vi "Begin.vi"(8 "error in":errorcluster) -> (0 "error out":errorcluster)   [LabVIEW 2015]
doc: "Called before other user functions, this VI is expected to open initial I/O refnums, load in file data, and do all program initialization. Notice that the <B>error out</B> terminal is simply used for data flow. Wiring it to other structures or subVIs ensures that this VI runs first."
uses:
  <vilib>/Rock Robotics/SystemInterfaces/DIO/FPGA_DIOPWMChannel.ctl
  <vilib>/Rock Robotics/WPI/SafetyOutput/WPI_SafetyOutputConfigMenu.ctl
  <vilib>/Rock Robotics/WPI/DriverStation/WPI_DriverStationRobotMode2.ctl
  <vilib>/Rock Robotics/WPI/Joystick/WPI_JoystickDeviceEnum.ctl
  <vilib>/Rock Robotics/WPI/CAN/TalonSRX/WPI_CANTalonSRX_APIControlMode.ctl
  <vilib>/Rock Robotics/WPI/CAN/TalonSRX/WPI_CANTalonSRX_BrakeOverride.ctl
  <vilib>/Rock Robotics/WPI/CAN/TalonSRX/WPI_CANTalonSRX_APIFeedbackSelect.ctl
  <vilib>/Rock Robotics/WPI/CAN/TalonSRX/WPI_CANTalonSRX_Params.ctl
  <vilib>/Rock Robotics/WPI/RobotDrive/WPI_RobotDriveOpen2MotorWithTalon.vi
  Robot Global Data.vi
  <vilib>/Rock Robotics/Network Tables/NT Write String Array.vi
  <vilib>/Rock Robotics/WPI/MotorControl/WPI_MotorControlOpenCANTalonSRX.vi
panel:
  in  "Reverse Feedback Sensor":bool
  in  "Reverse Closed-Loop Output":bool
  in  "Maximum Output Voltage":dbl=12.0
  in  "Reverse Limit Position":dbl=-50.0
  in  "Forward Limit Position":dbl=50.0
  in  "Encoder Codes Per Rev":u16=2122
  in  "D":dbl=10.0
  in  "I":dbl=0.0001
  in  "P":dbl=0.4
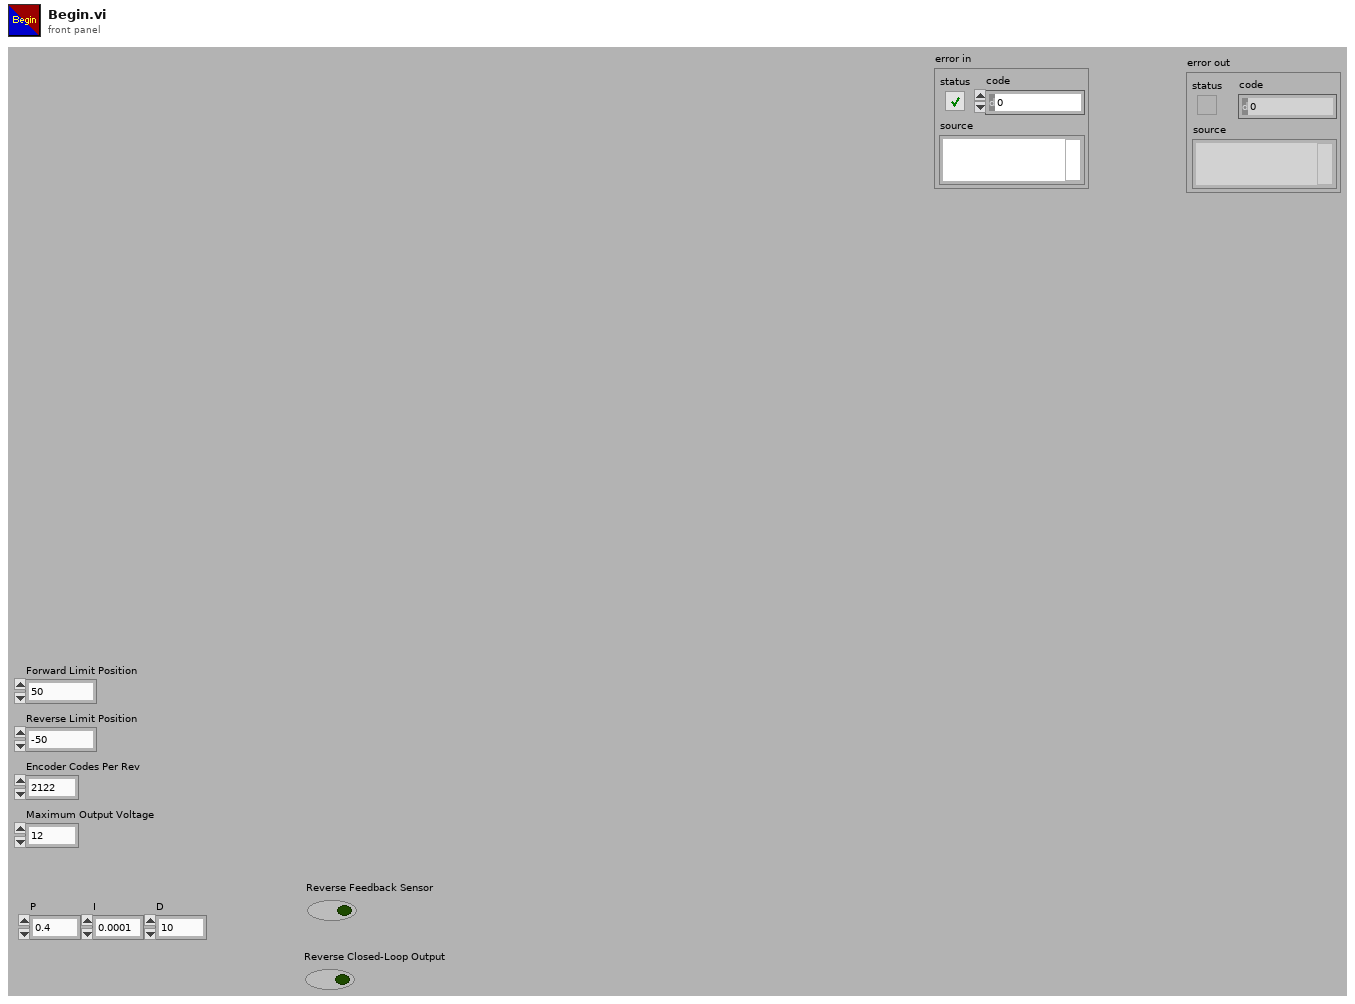
[diagram p1: front panel]
types:
  T1 = typedef "WPI_CANTalonSRX_APIControlMode.ctl" = enum8{"Percent VBus", "Speed", "Position", "Slave", "Unchanged / Invalid", "Voltage Compensation", "Current", "Motion Profile"}
  T2 = typedef "WPI_CANTalonSRX_Params.ctl" = u8
  T3 = typedef "WPI_CANTalonSRX_APIFeedbackSelect.ctl" = enum16{"Digital Quadrature Encoder", "Analog Potentiometer", "Analog Encoder", "Count on Quad-A (Rising-Edge)", "Count on Quad-A (Falling-Edge)", "CTR Magnetic Enc (Absolute)", "CTR Magnetic Enc (Relative)", "Pulse Width"}
  T4 = typedef "WPI_CANTalonSRX_BrakeOverride.ctl" = enum8{"No Override", "Override to Coast", "Override to Brake"}
  T5 = typedef "WPI_JoystickDeviceEnum.ctl" = enum16{"USB 0", "USB 1", "USB 2", "USB 3", "USB 4", "USB 5"}
  T6 = typedef "WPI_DriverStationRobotMode2.ctl" = enum16{"Autonomous Disabled", "Autonomous Enabled", "Teleop Disabled", "Teleop Enabled", "Disconnected", "Finish", "Test Disabled", "Test Enabled", "Emergency Stopped"}
  T7 = typedef "WPI_SafetyOutputConfigMenu.ctl" = enum16{"Enable", "Disable"}
  T8 = typedef "FPGA_DIOPWMChannel.ctl" = enum8{"PWM 0", "PWM 1", "PWM 2", "PWM 3", "PWM 4", "PWM 5", "PWM 6", "PWM 7", "PWM 8", "PWM 9", "PWM MXP 0", "PWM MXP 1", "PWM MXP 2", "PWM MXP 3", "PWM MXP 4", "PWM MXP 5", "PWM MXP 6", "PWM MXP 7", "PWM MXP 8", "PWM MXP 9", "Invalid"}
  T9 = typedef "WPI_MotorControlDeviceRef.ctl" = cluster{"DeviceStatus":errorcluster, "Type":T10, "PWM":cluster{"PWM Channel":T8, "DeadBand":T11}, "CAN":cluster{"Device Number":u8, "Control Mode":T12, "Semaphore":T13, "Max Vout":dbl, "TalonSRX Control Mode":T1}, "Invert":bool}
  T10 = typedef "WPI_MotorControlType.ctl" = enum16{"PWM", "CAN", "CANTalonSRX"}
  T11 = typedef "WPI_PWMDeadband.ctl" = cluster{"Name":string, "maxPositivePwm":i32, "minPositivePwm":i32, "centerPwm":i32, "maxNegativePwm":i32, "minNegativePwm":i32, "angularRange":u16}
  T12 = typedef "WPI_CANJaguar_ControlMode.ctl" = enum8{"Percent VBus", "Current", "Speed", "Position", "Voltage"}
  T13 = typedef "Semaphore RefNum" = refnum<k1>
  T14 = typedef "WPI_JoystickDevRef.ctl" = cluster{"Device":T5}
  T15 = typedef "WPI_RobotDriveDevRef.ctl" = cluster{"DevStatus":errorcluster, "Motors[]":T9[], "Square Inputs":bool, "Max Output":dbl}
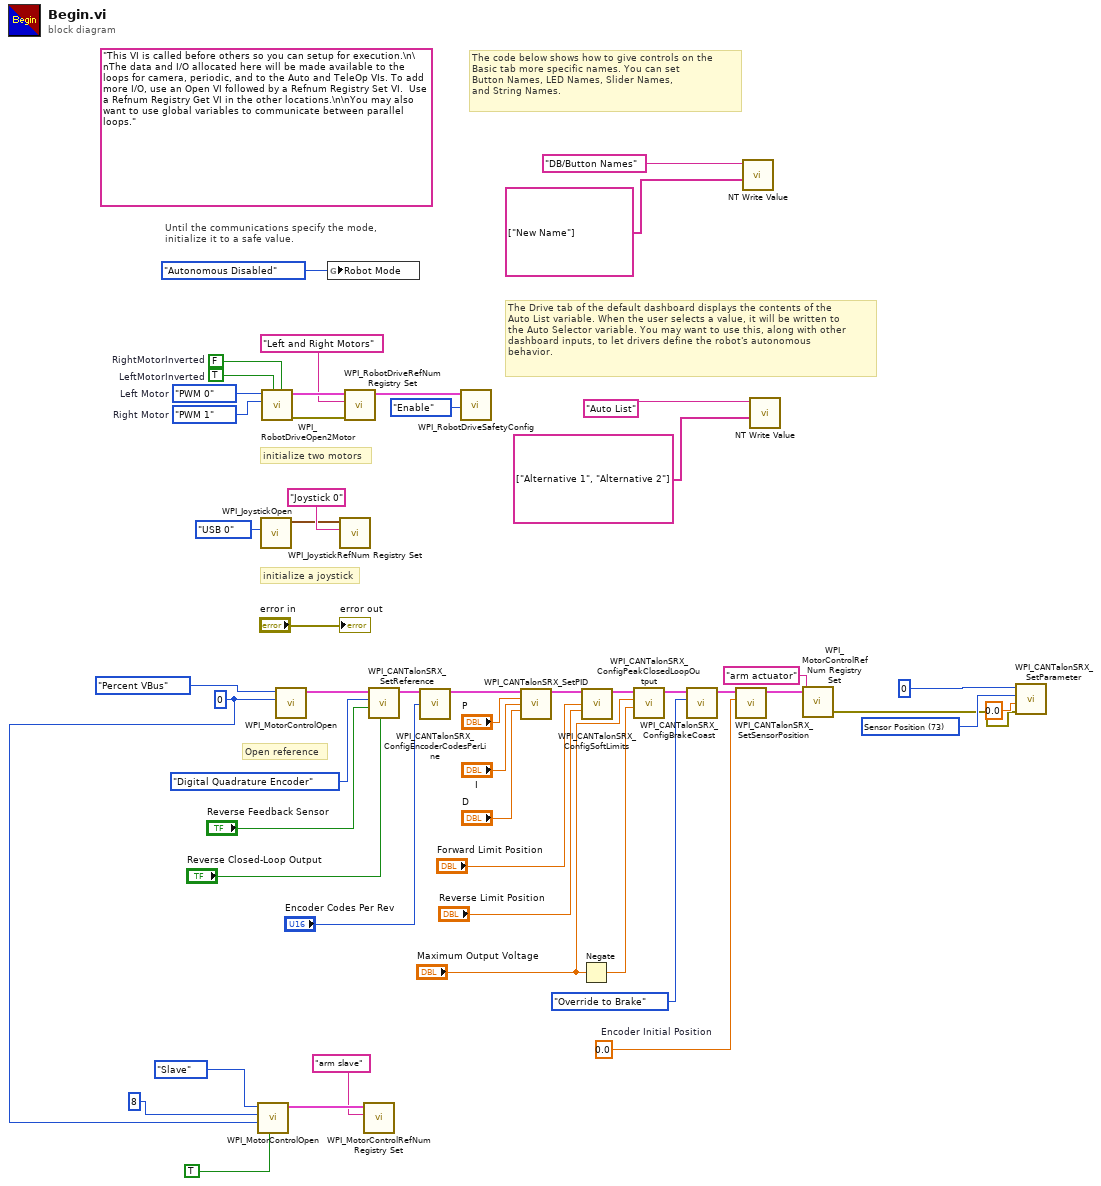
[diagram p0: block diagram]
diagram:
  w10 = T2 73 items=["Slot 0 - P"=1, "Slot 0 - I"=2, "Slot 0 - D"=3, "Slot 0 - F"=4, "Slot 0 - I Zone"=5, "Slot 0 - Ramp Rate"=6, "Slot 1 - P"=11, "Slot 1 - I"=12, "Slot 1 - D"=13, "Slot 1 - F"=14, "Slot 1 - I Zone"=15, "Slot 1 - Ramp Rate"=16, "Soft Limit - Forward"=21, "Soft Limit - Reverse"=22, "Soft Limit - Forward Enable"=23, "Soft Limit - Reverse Enable"=24, "On Boot - Brake Mode"=31, "On Boot - Limit Normally Closed - Forward"=32, "On Boot - Limit Normally Closed - Reverse"=33, "On Boot - Limit Disabled - Forward"=34, "On Boot - Limit Disabled - Reverse"=35, "Fault - Over Temp"=41, "Fault - Under Voltage"=42, "Fault - Forward Limit"=43, "Fault - Reverse Limit"=44, "Fault - Hardware Failure"=45, "Fault - Forward Soft Limit"=46, "Fault - Reverse Soft Limit"=47, "Sticky Fault - Over Temp"=48, "Sticky Fault - Under Voltage"=49, "Sticky Fault - Forward Limit"=50, "Sticky Fault - Reverse Limit"=51, "Sticky Fault - Forward Soft Limit"=52, "Sticky Fault - Reverse Soft Limit"=53, "Applied Throttle"=61, "Closed-Loop Error"=62, "Select Feedback Device"=63, "Reverse Closed-Loop Output"=64, "Mode Select"=65, "Profile Slot Select"=66, "Ramp Throttle"=67, "Reverse Feedback Sensor"=68, "Limit Switch Enabled"=69, "Limit Switch Closed - Forward"=70, "Limit Switch Closed - Reverse"=71, "Sensor Position"=73, "Sensor Velocity"=74, "Current"=75, "Brake is Enabled"=76, "Encoder Position"=77, "Encoder Velocity"=78, "Encoder Index Rise Events"=79, "Encoder A Pin State"=80, "Encoder B Pin State"=81, "Encoder Index Pin State"=82, "Analog In with Overflow"=83, "Analog In Velocity"=84, "Temperature"=85, "Battery Voltage"=86, "Reset Count"=87, "Reset Flags"=88, "Firmware Version"=89, "Settings Changed"=90, "Quad Filter Enable"=91, "Ignore Disable Broadcast"=92, "I Accumulator"=93, "Status 1 Frame Rate Ms"=94, "Status 2 Frame Rate Ms"=95, "Status 3 Frame Rate Ms"=96, "Status 4 Frame Rate Ms"=97, "Status 6 Frame Rate Ms"=98, "Status 7 Frame Rate Ms"=99, "Enable Index Pin Clear Position"=100, "Peak Positive Output"=104, "Nominal Positive Output"=105, "Peak Negative Output"=106, "Nominal Negative Output"=107, "Quad Index Pin Polarity"=108, "Status 8 Frame Rate Ms"=109, "Allow Position Overflow"=110, "Slot 0 - Allowable Closed-Loop Error"=111, "Number Potentiometer Turns"=112, "Encoder Codes Per Rev"=113, "Pulse Width Decoded Position"=114, "Analog Position"=115, "Voltage Compensation Rate (V/s)"=116, "Slot 1 - Allowable Closed-Loop Error"=117, "Motion Profile Has Underrun Err"=119] ("Parameter")
  w5 = u8 0 ("Device Number")
  w18 = 0.0  # Encoder Initial Position
  (unwired) "This VI is called before others so you can setup for execution.\n\nThe data and I/O allocated here will be made available to the loops for camera, periodic, and to the Auto and TeleOp VIs. To add more I/O, use an Open VI followed by a Refnum Registry Set VI.  Use a Refnum Registry Get VI in the other locations.\n\nYou may also want to use global variables to communicate between parallel loops."
  w45 = FPGA_DIOPWMChannel."PWM 1"  # Right Motor
  w46 = FPGA_DIOPWMChannel."PWM 0"  # Left Motor
  w50 = TRUE  # LeftMotorInverted
  w51 = FALSE  # RightMotorInverted
  # "Open reference"
  # "The Drive tab of the default dashboard displays the contents of the\nAuto List variable. When the user selects a value, it will be written to\nthe Auto Selector variable. You may want to use this, along with other\ndashboard inputs, to let drivers define the robot's autonomous\nbehavior."
  # "The code below shows how to give controls on the\nBasic tab more specific names. You can set\nButton Names, LED Names, Slider Names,\nand String Names."
  # "initialize a joystick"
  # "Until the communications specify the mode,\ninitialize it to a safe value."
  # "initialize two motors"
  n1 = call-poly <vilib>:"WPI_MotorControlOpen.vi"("Invert"=TRUE, "Master Device Number"=w5, "Device Number"=u8 8, "Control Mode"=WPI_CANTalonSRX_APIControlMode."Slave") -> ("MotorControlDeviceRef"=w2:T9)  [unwired: 1 in, 6 out]
  n2 = call <vilib>:"WPI_JoystickOpen.vi"("JoystickDevice"=WPI_JoystickDeviceEnum."USB 0") -> ("JoystickDevRef"=w40:T14)  [unwired: 10 in]
  n3 = call-poly <vilib>:"WPI_RobotDriveOpen2Motor.vi"("Right Motor Inverted"=w51, "Left Motor Inverted"=w50, "Right Motor"=w45, "Left Motor"=w46) -> ("error out"=w47:errorcluster, "RobotDriveDevRef"=w49:T15)  [unwired: 1 in, 5 out]
  n4 = call-poly <vilib>:"WPI_MotorControlOpen.vi"("Device Number"=w5, "Control Mode"=WPI_CANTalonSRX_APIControlMode."Percent VBus") -> ("MotorControlDeviceRef"=w17:T9)  [unwired: 3 in, 6 out]
  n5 = global write "Robot Global Data.vi" "Robot Mode"(WPI_DriverStationRobotMode2."Autonomous Disabled" ("Robot Mode")) -> ()
  n6 = call <vilib>:"WPI_JoystickRefNum Registry Set.vi"("refnum name"="Joystick 0", "JoystickDevRef"=w40) -> ()  [unwired: 8 in, 2 out]
  n7 = call <vilib>:"WPI_RobotDriveRefNum Registry Set.vi"("error in (no error)"=w47, "refnum name"="Left and Right Motors", "RobotDriveDevRef"=w49) -> ("RobotDriveDevRef"=w44:T15)  [unwired: 1 in, 7 out]
  n8 = call <vilib>:"WPI_MotorControlRefNum Registry Set.vi"("refnum name"="arm slave", "MotorControlDevRef"=w2) -> ()  [unwired: 8 in, 2 out]
  n9 = call <vilib>:"WPI_CANTalonSRX_SetReference.vi"("Reverse Closed-Loop Output"="Reverse Closed-Loop Output", "Reverse Feedback Sensor"="Reverse Feedback Sensor", "Feedback Reference"=WPI_CANTalonSRX_APIFeedbackSelect."Digital Quadrature Encoder", "CAN Talon SRX Ref"=w17) -> ("CAN Talon SRX Ref"=w16:T9)  [unwired: 6 in, 1 out]
  n10 = call <vilib>:"WPI_CANTalonSRX_ConfigEncoderCodesPerLine.vi"("CAN Talon SRX Ref"=w16, "Number Encoder Lines\n(Counts Per Rotation)"="Encoder Codes Per Rev") -> ("CAN Talon SRX Ref"=w27:T9)  [unwired: 12 in, 1 out]
  n11 = call <vilib>:"WPI_RobotDriveSafetyConfig.vi"("mode"=WPI_SafetyOutputConfigMenu."Enable", "RobotDriveDevRef"=w44) -> ()  [unwired: 8 in, 2 out]
  n12 = call <vilib>:"WPI_CANTalonSRX_SetPID.vi"("CAN Talon SRX Ref"=w27, "P"="P", "I"="I", "D"="D") -> ("CAN Talon SRX Ref"=w26:T9)  [unwired: 10 in, 1 out]
  n13 = Negate(x="Maximum Output Voltage") -> (-x=w13:dbl)
  n14 = call <vilib>:"WPI_CANTalonSRX_ConfigSoftLimits.vi"("CAN Talon SRX Ref"=w26, "Forward Limit Position"="Forward Limit Position", "Reverse Limit Position"="Reverse Limit Position") -> ("CAN Talon SRX Ref"=w23:T9)  [unwired: 11 in, 1 out]
  n15 = call <vilib>:"WPI_CANTalonSRX_ConfigPeakClosedLoopOutput.vi"("Reverse Peak Output"=w13, "Forward Peak Output"="Maximum Output Voltage", "CAN Talon SRX Ref"=w23) -> ("CAN Talon SRX Ref"=w21:T9)  [unwired: 7 in, 1 out]
  n16 = call <vilib>:"WPI_CANTalonSRX_ConfigBrakeCoast.vi"("Brake / Coast Mode"=WPI_CANTalonSRX_BrakeOverride."Override to Brake", "CAN Talon SRX Ref"=w21) -> ("CAN Talon SRX Ref"=w19:T9)  [unwired: 8 in, 1 out]
  n17 = call <vilib>:"WPI_CANTalonSRX_SetSensorPosition.vi"("New Sensor Position"=w18, "CAN Talon SRX Ref"=w19) -> ("CAN Talon SRX Ref"=w12:T9)  [unwired: 8 in, 1 out]
  n18 = call-poly <vilib>:"NT Write Value.vi"("String Array"=string[] ["New Name"], "Name"="DB/Button Names") -> ()  [unwired: 9 in, 1 out]
  n19 = call-poly <vilib>:"NT Write Value.vi"("String Array"=string[] ["Alternative 1", "Alternative 2"], "Name"="Auto List") -> ()  [unwired: 9 in, 1 out]
  n20 = call <vilib>:"WPI_MotorControlRefNum Registry Set.vi"("refnum name"="arm actuator", "MotorControlDevRef"=w12) -> ("error out"=w8:errorcluster)  [unwired: 8 in, 1 out]
  n21 = call <vilib>:"WPI_CANTalonSRX_SetParameter.vi"("error in (no error)"=w8, "Value"=0.0, "Parameter"=w10, "Device ID (0)"=u8 0) -> ()  [unwired: 6 in, 2 out]
  "error out" <- "error in"
